vi "Dialogue_TwoButton.vi"(4 "Btn_2 Text":string="Cancel", 6 "Btn_1 Text":string="OK", 8 "error in":errorcluster, 10 "Message":string, 11 "Title":string) -> (0 "error out":errorcluster, 2 "Btn_2?":bool=TRUE, 3 "Btn_1?":bool=TRUE)   [LabVIEW 2020, in "hse-ui.lvlib"]
doc: "Shows a dialog window with a message and two buttons (default: \"Ok\" and \"Cancel\")\n\n____\nHAMPEL SOFTWARE ENGINEERING v3.8.0 (2023-12-18 14:41)"
uses:
  hse-ui.lvlib
  FPControl/FPControl_Actions.ctl
panel:
  in  "Btn_Cancel":bool
  in  "Btn_OK":bool
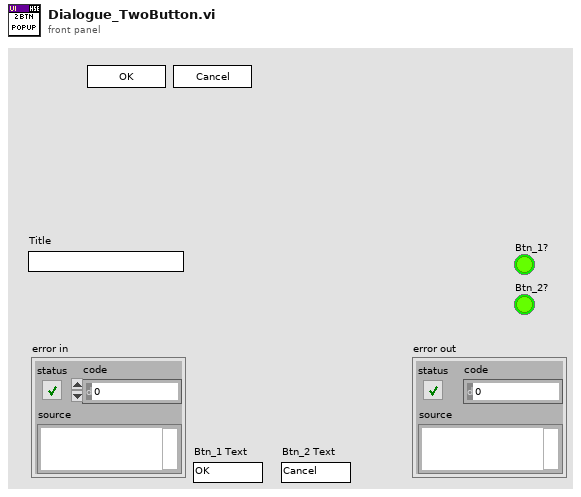
[diagram p1: front panel]
types:
  T1 = typedef "hse-ui.lvlib/FPControl_Actions.ctl" = enum16{"Open", "Hide", "Close", "Bring To Front", "Center", "Minimize", "Maximize"}
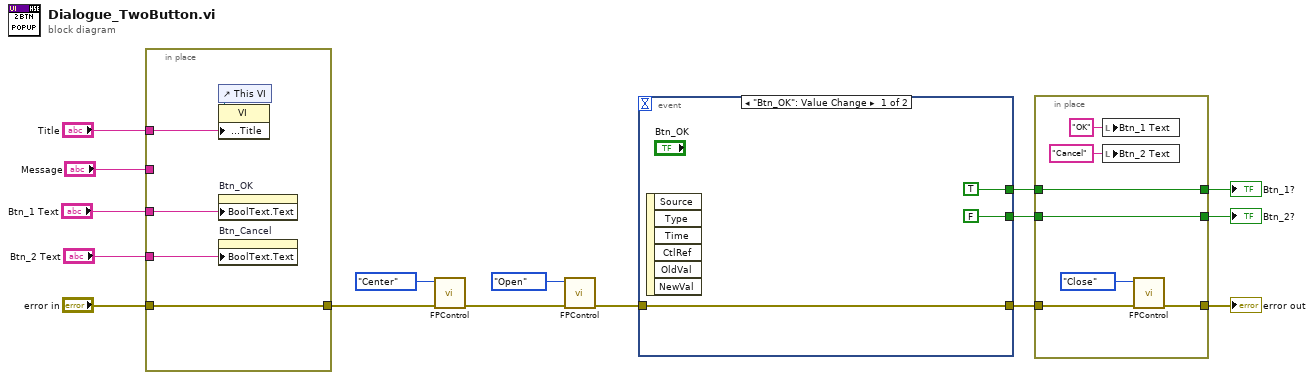
[diagram p0: block diagram]
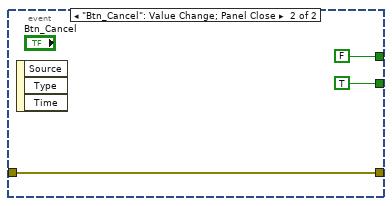
[diagram p2: hidden frame]
diagram:
  n1 = in-place {
    in-place-border: "error in" -> [w21]
    in-place-border: [w21] -> w10
    in-place-border: "Title" -> [w19]
    in-place-border: "Message" -> [_]
    in-place-border: "Btn_1 Text" -> [w18]
    in-place-border: "Btn_2 Text" -> [w17]
    n2 = control-ref of="This VI"() -> (w20:refnum<vi>)
    n3 = property class="VI"(reference=w20, "Front Panel.Title"=w19) -> ()  [unwired: 1 in, 2 out]
    n4 = property on="Btn_OK" class="Bool"("BoolText.Text"=w18) -> ()  [unwired: 2 in, 2 out]
    n5 = property on="Btn_Cancel" class="Bool"("BoolText.Text"=w17) -> ()  [unwired: 2 in, 2 out]
  }
  n6 = call "FPControl.vi"("error in"=w10, "Function"=FPControl_Actions."Center") -> ("error out"=w14:errorcluster)  [unwired: 9 out]
  n7 = call "FPControl.vi"("error in"=w14, "Function"=FPControl_Actions."Open") -> ("error out"=w8:errorcluster)  [unwired: 9 out]
  n8 = event shown="[0] \"Btn_OK\": Value Change" {
    selector: _ -> [_ _]
    dyn-events: _ -> [_ _]
    timeout: _ -> [_ _]
    tunnel: w8 -> [w24 w27]
    tunnel: [w24 w27] -> w12
    tunnel: [TRUE FALSE] -> w4
    tunnel: [FALSE TRUE] -> w3
    event "Btn_OK": Value Change {
      n9 = event-data() -> ()  [unwired: 1 in, 6 out]
    }
    event "Btn_Cancel": Value Change; Panel Close {
      n10 = event-data() -> ()  [unwired: 1 in, 3 out]
    }
  }
  n11 = in-place {
    in-place-border: [w33] -> w13
    in-place-border: w12 -> [w32]
    in-place-border: w4 -> [w29]
    in-place-border: w3 -> [w28]
    in-place-border: [w29] -> w2
    in-place-border: [w28] -> w1
    n12 = local write "Btn_1 Text"("OK" ("Btn_1 Text")) -> ()
    n13 = local write "Btn_2 Text"("Cancel" ("Btn_1 Text")) -> ()
    n14 = call "FPControl.vi"("error in"=w32, "Function"=FPControl_Actions."Close") -> ("error out"=w33:errorcluster)  [unwired: 9 out]
  }
  "error out" <- w13
  "Btn_1?" <- w2
  "Btn_2?" <- w1
